vi "sv_Build Unit Label (octave info).vi"(8 "error in (no error)":errorcluster, 9 "octave info":T1={"standard"=enum."ANSI S1.11", "bandwidth"=enum."1 octave", "low band"=0, "high band"=0, "weighting filter"=0, "dB reference"=0.0, "dB On"=FALSE, "unit label"="", "channel name"="", "description"="", "engineering units"=1, "custom label"="", "spectrum type"=enum."magnitude", "spectral density"=FALSE, "filters settled"=FALSE} {"engineering units" items=["custom..."=0, "V"=1, "A"=21, "C"=30, "pC"=31, "s"=32, "-"=29, "Pa"=2, "N"=20, "g"=3, "m/s^2"=4, "m/s"=5, "m"=6, "mm/s"=12, "mm"=13, "micron/s"=14, "micron"=15, "in/s^2"=7, "in/s"=8, "in"=9, "mil/s"=10, "mil"=11, "rad/s^2"=16, "rad/s"=17, "rad"=18, "deg/s^2"=26, "deg/s"=27, "deg"=28, "RPM"=22, "cycle/s^2"=23, "Hz"=24, "cycle"=25, "strain"=19]; "dB reference" format="%.2e"; "weighting filter" items=["Linear", "A-weighting", "B-weighting", "C-weighting", "ITU-R 468-4", "Dolby", "CCITT", "C-message", "Wb", "Wc", "Wd", "We", "Wf", "Wh", "Wj", "Wk", "Wm", "AES17 20 kHz lowpass", "AES17 40 kHz lowpass", "AES17 20 kHz highpass", "AES17 40 kHz highpass"]}) -> (0 "error out":errorcluster, 1 "octave info out":T1={"standard"=enum."ANSI S1.11", "bandwidth"=enum."1 octave", "low band"=0, "high band"=0, "weighting filter"=0, "dB reference"=0.0, "dB On"=FALSE, "unit label"="", "channel name"="", "description"="", "engineering units"=1, "custom label"="", "spectrum type"=enum."magnitude", "spectral density"=FALSE, "filters settled"=FALSE} {"engineering units" items=["custom..."=0, "V"=1, "A"=21, "C"=30, "pC"=31, "s"=32, "-"=29, "Pa"=2, "N"=20, "g"=3, "m/s^2"=4, "m/s"=5, "m"=6, "mm/s"=12, "mm"=13, "micron/s"=14, "micron"=15, "in/s^2"=7, "in/s"=8, "in"=9, "mil/s"=10, "mil"=11, "rad/s^2"=16, "rad/s"=17, "rad"=18, "deg/s^2"=26, "deg/s"=27, "deg"=28, "RPM"=22, "cycle/s^2"=23, "Hz"=24, "cycle"=25, "strain"=19]; "dB reference" format="%.2e"; "weighting filter" items=["Linear", "A-weighting", "B-weighting", "C-weighting", "ITU-R 468-4", "Dolby", "CCITT", "C-message", "Wb", "Wc", "Wd", "We", "Wf", "Wh", "Wj", "Wk", "Wm", "AES17 20 kHz lowpass", "AES17 40 kHz lowpass", "AES17 20 kHz highpass", "AES17 40 kHz highpass"]}, 2 "unit label":string)   [LabVIEW 2017, in "SoundVib_Octave_2014 standard.lvlib"]
uses:
  <vilib>/addons/Sound and Vibration/svt_Octave/SoundVib_Octave_2014 standard.lvlib
  <vilib>/addons/_NISVFA/_Shared subVIs/Controls/svc_Octave Info.ctl
  <vilib>/addons/_NISVFA/_Shared subVIs/Controls/svc_Octave Standard.ctl
  <vilib>/addons/_NISVFA/_Shared subVIs/Controls/svc_Weighting Filter Text Ring.ctl
  <vilib>/addons/_NISVFA/_Shared subVIs/Controls/svc_Engineering Units Text Ring.ctl
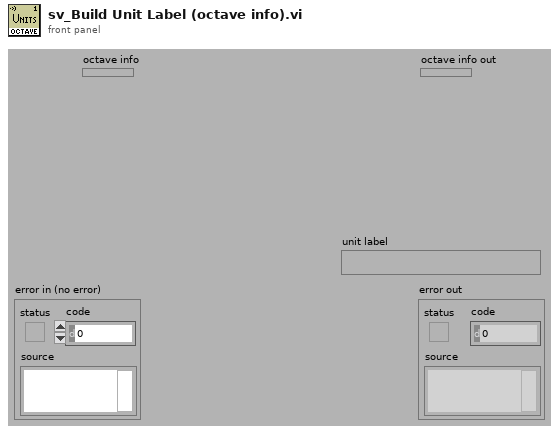
[diagram p1: front panel]
types:
  T1 = typedef "svc_Octave Info.ctl" = cluster{"standard":T2, "bandwidth":enum16{"1 octave", "1/3 octave", "1/6 octave", "1/12 octave", "1/24 octave"}, "low band":i32, "high band":i32, "weighting filter":T3, "dB reference":dbl, "dB On":bool, "unit label":string, "channel name":string, "description":string, "engineering units":T4, "custom label":string, "spectrum type":enum16{"power", "magnitude"}, "spectral density":bool, "filters settled":bool}
  T2 = typedef "svc_Octave Standard.ctl" = enum16{"ANSI S1.11", "IEC 61260"}
  T3 = typedef "svc_Weighting Filter Text Ring.ctl" = u16
  T4 = typedef "svc_Engineering Units Text Ring.ctl" = u16
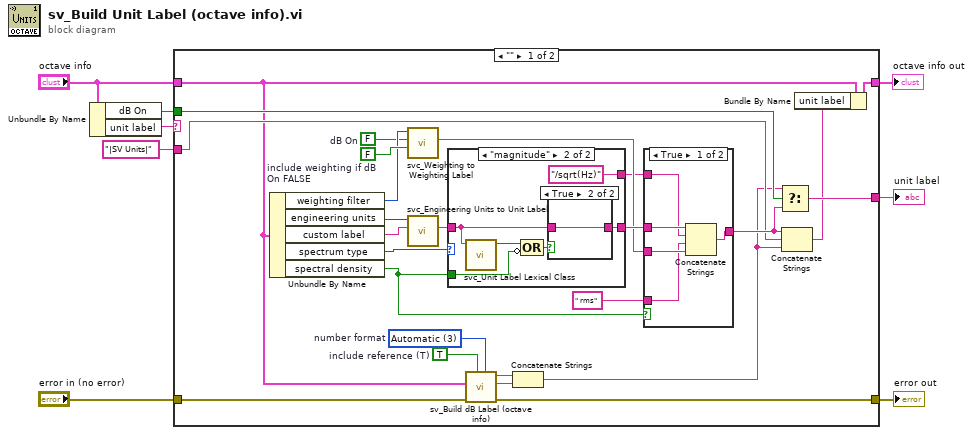
[diagram p0: block diagram]
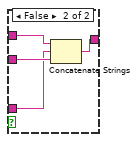
[diagram p2: hidden frame]
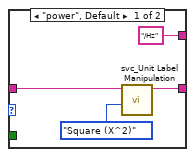
[diagram p3: hidden frame]
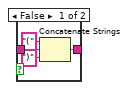
[diagram p4: hidden frame]
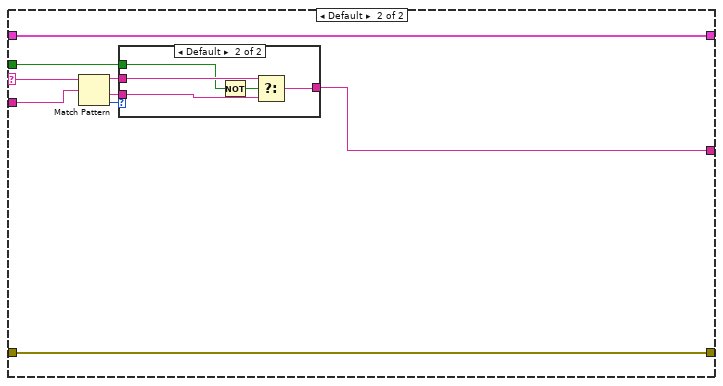
[diagram p5: hidden frame]
diagram:
  n1 = Unbundle By Name("octave info") -> ("dB On"=w2:bool, "unit label"=w4:string)
  n2 = case shown="\"\"" w4 {
    selector: w4 -> [_ w64]
    tunnel: [w17 w61] -> w8
    tunnel: "octave info" -> [w9 w61]
    tunnel: "error in (no error)" -> [w18 w59]
    tunnel: [w14 w59] -> w5
    tunnel: "|SV Units|" ("string") -> [w12 w63]
    tunnel: w2 -> [w16 w62]
    tunnel: [w15 w60] -> w1
    frame "" {
      w30 = TRUE  # include reference (T)
      w34 = FALSE  # include weighting if dB On FALSE
      w19 = FALSE  # dB On
      w33 = i16 3 items=["Engineering", "Exponential", "Fractional", "Automatic"]  # number format
      n3 = Unbundle By Name(w9) -> ("weighting filter"=w23:T3, "engineering units"=w26:T4, "custom label"=w25:string, "spectrum type"=w27:enum16{"power", "magnitude"}, "spectral density"=w20:bool)
      n4 = call <vilib>:"svc_Weighting to Weighting Label.vi"("include weighting if dB On False (T)"=w34, "dB On (T)"=w19, "weighting filter"=w23) -> ("weighting string"=w28:string)  [unwired: 7 in, 1 out]
      n5 = call <vilib>:"svc_Engineering Units to Unit Label.vi"("custom label"=w25, "engineering units"=w26) -> ("unit label"=w24:string)  [unwired: 8 in, 1 out]
      n6 = case shown="\"magnitude\"" w27 {
        tunnel: w24 -> [w46 w51]
        tunnel: [w45 w50] -> w29
        tunnel: ["/Hz" "/sqrt(Hz)"] -> w21
        tunnel: w20 -> [_ w48]
        frame "power", Default {
          n7 = call <vilib>:"svc_Unit Label Manipulation.vi"("operation"=enum16{"Square (X^2)", "Divide (X/Y)"}."Square (X^2)", "X unit label"=w46) -> ("resulting unit label"=w45:string)  [unwired: 5 in]
        }
        frame "magnitude" {
          n8 = call <vilib>:"svc_Unit Label Lexical Class.vi"("unit label"=w51) -> ("letters only?"=w52:bool)  [unwired: 6 in]
          n9 = Compound Arithmetic op=OR(w52, invert w48) -> (w49:bool)
          n10 = case shown="True" w49 {
            tunnel: w51 -> [w57 w58]
            tunnel: [w56 w58] -> w50
            frame False {
              n11 = Concatenate Strings("(" ("string"), w57, ")" ("string")) -> (w56:string)
            }
            frame True {
            }
          }
        }
      }
      n12 = call <vilib>:"sv_Build dB Label (octave info).vi"("number format"=w33, "include reference (T)"=w30, "error in (no error)"=w18, "octave info"=w9) -> ("error out"=w14:errorcluster, "ref label"=w32:string, "dB( )"=w31:string)  [unwired: 4 in, 1 out]
      n13 = Concatenate Strings(w31, w32) -> (w11:string)
      n14 = case shown="True" w20 {
        tunnel: w29 -> [w39 w43]
        tunnel: [w38 w42] -> w13
        tunnel: w28 -> [w37 w41]
        tunnel: " rms" -> [w36 w40]
        tunnel: w21 -> [w35 _]
        frame True {
          n15 = Concatenate Strings(w39, w35, w36, w37) -> (w38:string)
        }
        frame False {
          n16 = Concatenate Strings(w43, w40, w41) -> (w42:string)
        }
      }
      n17 = Select(t=w11, s=w16, f=w13) -> (s? t:f=w15:string)
      n18 = Concatenate Strings(w13, w12, w11) -> (w10:string)
      n19 = Bundle By Name(cluster=w9, "unit label"=w10) -> (w17:T1)
    }
    frame Default {
      n20 = Match Pattern(string=w64, regular expression=w63) -> (before substring=w67:string, after substring=w66:string, offset past match=w65:i32)  [unwired: 1 in, 1 out]
      n21 = case shown="Default" w65 {
        tunnel: w67 -> [w68 w73]
        tunnel: w66 -> [_ w72]
        tunnel: [w68 w71] -> w60
        tunnel: w62 -> [_ w70]
        frame -1 {
        }
        frame Default {
          n22 = Not(x=w70) -> (.not. x?=w69:bool)
          n23 = Select(t=w73, s=w69, f=w72) -> (s? t:f=w71:string)
        }
      }
    }
  }
  "octave info out" <- w8
  "unit label" <- w1
  "error out" <- w5
